vi "Create Trigger.vi"(6 "This VI":refnum<vi>, 8 "error in (no error)":errorcluster) -> (0 "error out":errorcluster)   [LabVIEW 2014, in "Waveform-Processing-Custom-Device Engine.lvlib" / "Inline Async API.lvlib"]
uses:
  Inline Async API.lvlib
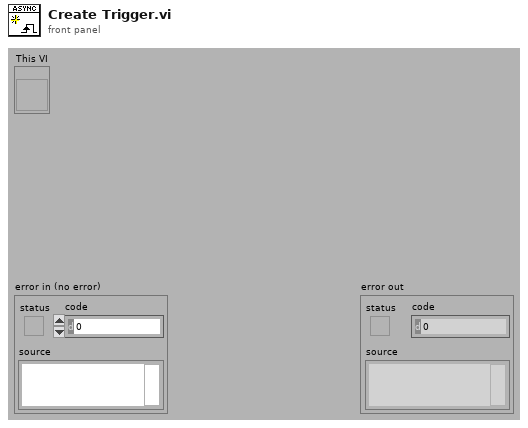
[diagram p1: front panel]
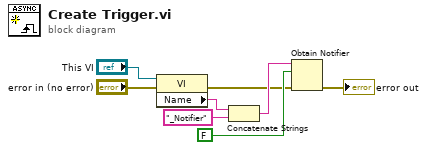
[diagram p0: block diagram]
diagram:
  n1 = property class="VI"(reference="This VI", error in="error in (no error)") -> (error out=w1:errorcluster, "Name"=w5:string)  [unwired: 1 out]
  n2 = Concatenate Strings(w5, "_Notifier" ("name (unnamed)")) -> (w3:string)
  n3 = Obtain Notifier(name (unnamed)=w3, notification data type=FALSE, error in (no error)=w1) -> (error out=→"error out":errorcluster)  [unwired: 1 in, 2 out]
